vi "testDBL Data Arrays Within Delta.vi"(8 "error in (no error)":errorcluster, 11 "TestCase in":refnum<class "1D Array Test Case.lvclass">) -> (0 "error out":errorcluster, 3 "TestCase out":refnum<class "1D Array Test Case.lvclass">)   [LabVIEW 2015, in "1D Array Test Case.lvclass"]
uses:
  1D Array Test Case.lvclass
  <vilib>/addons/_JKI Toolkits/VI Tester/TestCase.llb/TestCase.lvclass
  VITAC.lvlib
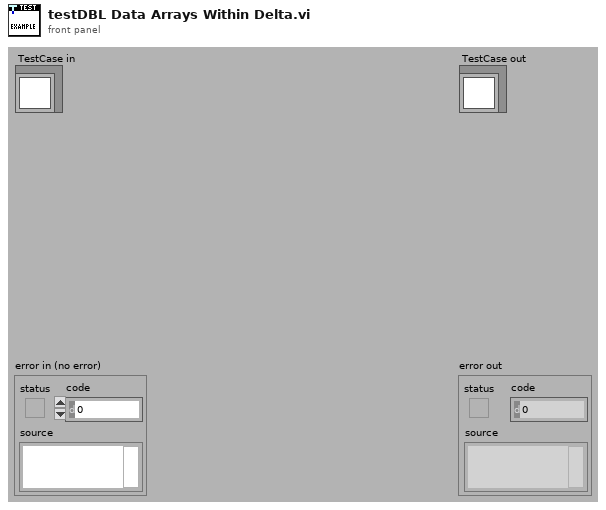
[diagram p1: front panel]
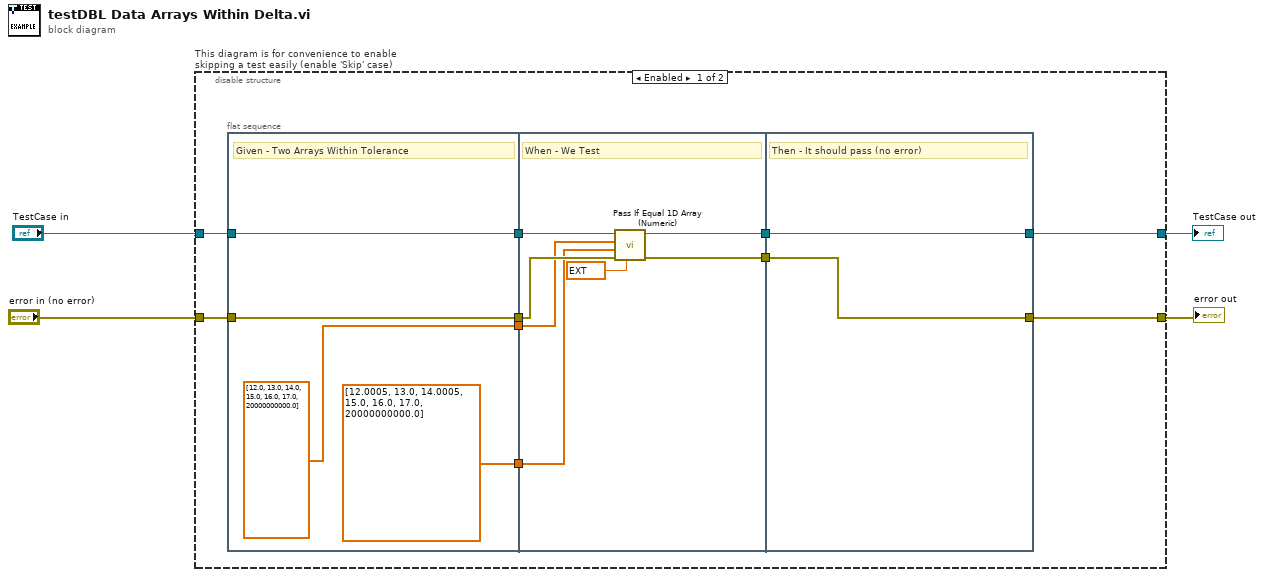
[diagram p0: block diagram]
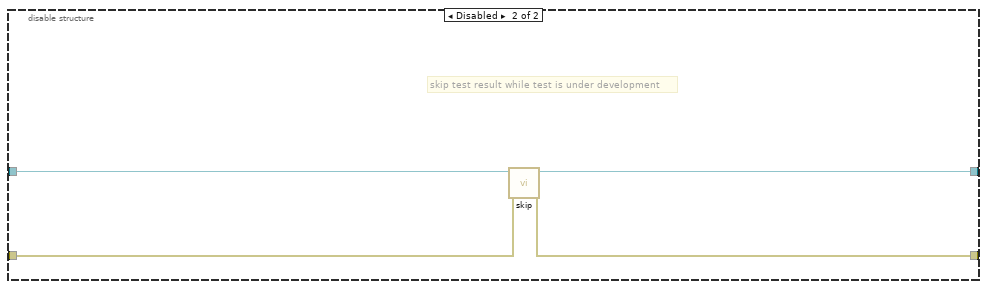
[diagram p2: hidden frame]
diagram:
  n1 = disable-structure "This diagram is for convenience to enable skipping a test easily (enable 'Skip' case)" shown="Enabled" {
    disable-tunnel: "TestCase in" -> [w13 w31]
    disable-tunnel: [w12 w29] -> w1
    disable-tunnel: [w8 w30] -> w3
    disable-tunnel: "error in (no error)" -> [w9 w28]
    frame Enabled {
      n2 = flat-sequence {
        tunnel: [w18] -> w14
        tunnel: w13 -> [w18]
        tunnel: [w17] -> w10
        tunnel: w9 -> [w17]
        tunnel: [dbl[] [12.0, 13.0, 14.0, 15.0, 16.0, 17.0, 20000000000.0] ("x")] -> w6
        tunnel: [dbl[] [12.0005, 13.0, 14.0005, 15.0, 16.0, 17.0, 20000000000.0] ("x")] -> w5
        tunnel: w14 -> [w25]
        tunnel: [w24] -> w11
        tunnel: w10 -> [w23]
        tunnel: [w22] -> w7
        tunnel: w6 -> [w20]
        tunnel: w5 -> [w19]
        tunnel: [w27] -> w12
        tunnel: w11 -> [w27]
        tunnel: [w26] -> w8
        tunnel: w7 -> [w26]
        frame #0 {
          # "Given - Two Arrays Within Tolerance"
        }
        frame #1 {
          # "When - We Test"
          n3 = call "Pass If Equal 1D Array (Numeric).vi"("delta (optional)"=ext 0.0006, "error in (no error)"=w23, "actual"=w19, "expected"=w20, "TestCase in"=w25) -> ("error out"=w22:errorcluster, "TestCase out"=w24:refnum<class "1D Array Test Case.lvclass">)  [unwired: 5 in]
        }
        frame #2 {
          # "Then - It should pass (no error)"
        }
      }
    }
    frame Disabled {
      # "skip test result while test is under development"
      n4 = call <vilib>:"skip.vi"("error in (no error)"=w28, "TestCase in"=w31) -> ("error out"=w30:errorcluster, "TestCase out"=w29:refnum<class "1D Array Test Case.lvclass">)  [unwired: 8 in]
    }
  }
  "error out" <- w3
  "TestCase out" <- w1
